vi "GP1 get pressure.vi"(3 "error in":errorcluster) -> (0 "error out":errorcluster, 1 "Baratron (Torr)":dbl, 2 "Actual (psi)":dbl)   [LabVIEW 2013, in "GP1.lvclass"]
uses:
  GP1.lvclass
  <vilib>/DAQmx/read.llb/DAQmx Read (Analog DBL 1Chan 1Samp).vi
  <vilib>/DAQmx/read.llb/DAQmx Read (Analog 1D DBL 1Chan NSamp).vi
  <vilib>/Analysis/baseanly.llb/Mean (DBL).vi
  <vilib>/DAQmx/miscellaneous.llb/DAQmx Fill In Error Info.vi
  <vilib>/Analysis/NI_AALBase.lvlib
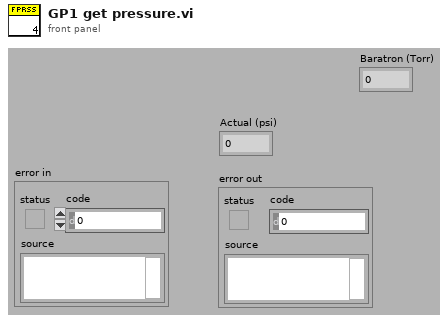
[diagram p1: front panel]
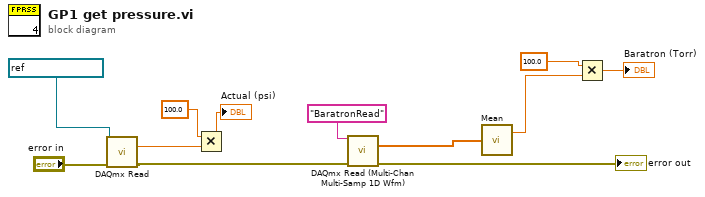
[diagram p0: block diagram]
diagram:
  n1 = call-poly <vilib>:"DAQmx Read.vi"("task/channels in"=refnum<k21> "pressureread" ("readtask"), "error in"="error in") -> ("data"=w11:dbl, "error out"=w6:errorcluster)  [unwired: 12 out]
  n2 = Multiply(x=100.0 ("y"), y=w11) -> (x*y=→"Actual (psi)":dbl)
  n3 = call-poly "DAQmx Read (Multi-Chan Multi-Samp 1D Wfm).vi"("task/channels in"="BaratronRead" ("new task name"), "error in"=w6) -> ("data"=w4:dbl[], "error out"=→"error out":errorcluster)  [unwired: 2 in, 10 out]
  n4 = call-poly <vilib>:"Mean.vi"("X"=w4) -> ("mean"=w2:dbl)  [unwired: 1 out]
  n5 = Multiply(x=100.0 ("y"), y=w2) -> (x*y=→"Baratron (Torr)":dbl)
